vi "Charge_then_Discharge.vi"() -> ()   [LabVIEW 2020]
panel:
  out "PS error out":errorcluster
  out "PS Visa Out":refnum<visa-resource-name>
  in  "Discharge Current Cutoff":dbl
  in  "Discharge Current Setpoint (A)":dbl format="%#.6g"
  in  "Wait time":dbl
  in  "Batteryname":string
  in  "Charge Current Cutoff":dbl
  in  "Charge Current  Setpoint (A)":dbl format="%#.6g"
  in  "Battery Select":T1(ring)
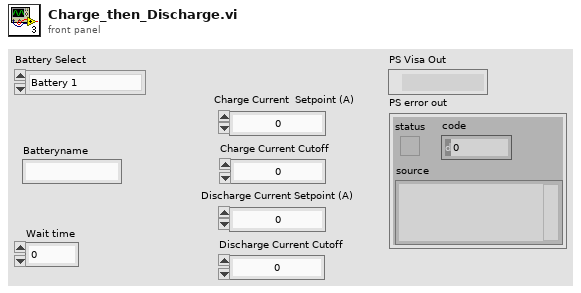
[diagram p1: front panel]
types:
  T1 = enum16{"Battery 1", "Battery 2", "Battery 3", "Battery 1&2", "Battery 1&3", "Battery 2&3", "Battery 1&2&3"}
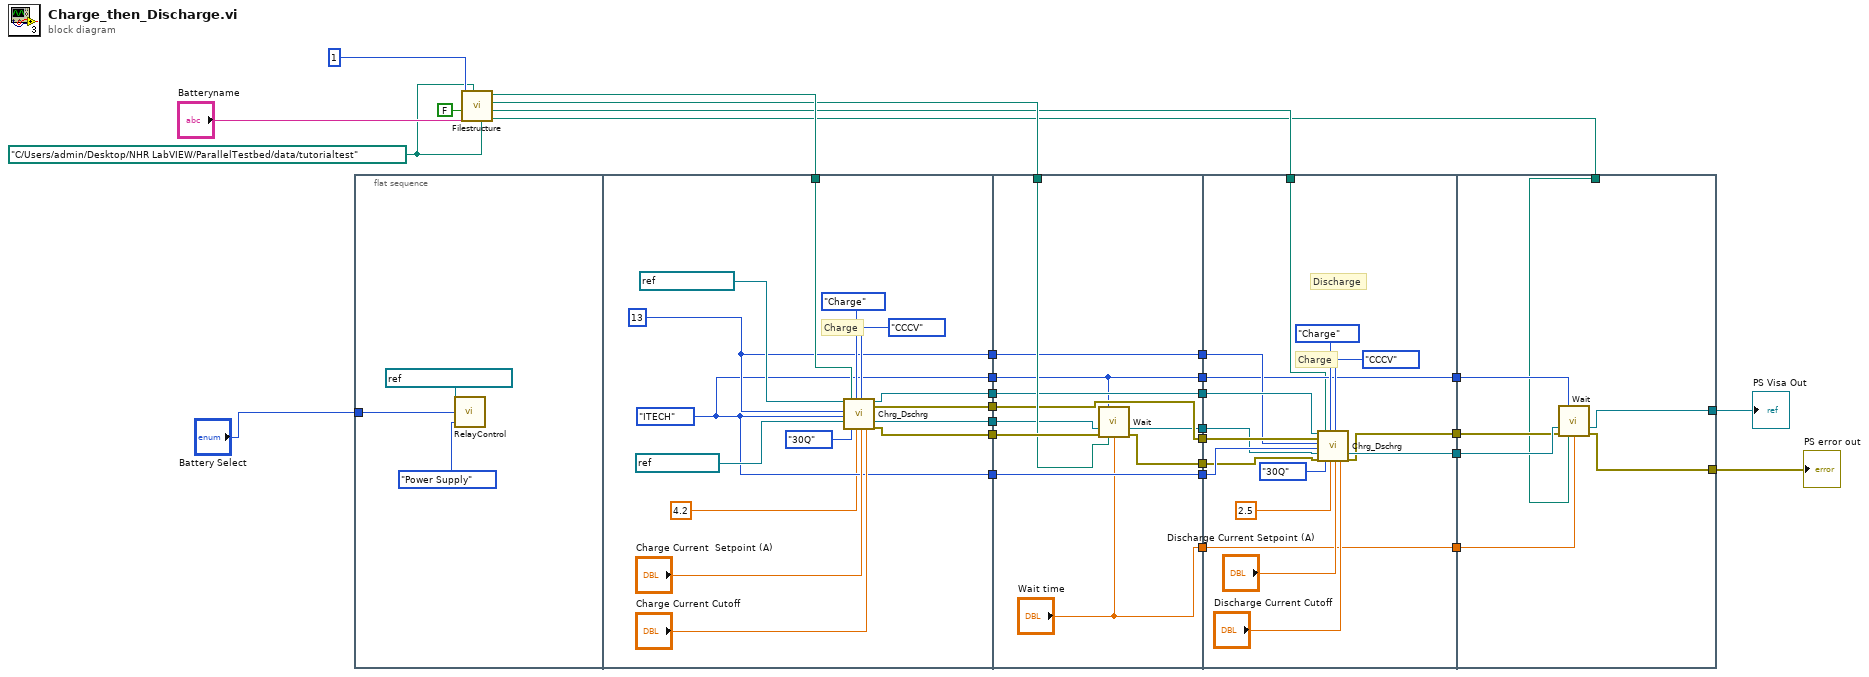
[diagram p0: block diagram]
diagram:
  w26 = path "C:/Users/admin/Desktop/NHR LabVIEW/ParallelTestbed/data/tutorialtest" ("Discharge filepath")
  n1 = flat-sequence {
    tunnel: "Battery Select" -> [w31]
    tunnel: w25 -> [w44]
    tunnel: [w41] -> w24
    tunnel: [w36] -> w23
    tunnel: [w38] -> w21
    tunnel: [w39] -> w19
    tunnel: [w37] -> w17
    tunnel: [w36] -> w15
    tunnel: [w35] -> w11
    tunnel: w24 -> [w59]
    tunnel: w23 -> [w50]
    tunnel: w22 -> [w58]
    tunnel: w21 -> [w57]
    tunnel: [w57] -> w20
    tunnel: w19 -> [w56]
    tunnel: [w56] -> w18
    tunnel: w17 -> [w55]
    tunnel: [w55] -> w16
    tunnel: w15 -> [w54]
    tunnel: [w54] -> w14
    tunnel: [w53] -> w13
    tunnel: [w52] -> w12
    tunnel: w11 -> [w51]
    tunnel: [w50] -> w8
    tunnel: ["Wait time"] -> w4
    tunnel: w20 -> [w73]
    tunnel: w18 -> [w72]
    tunnel: w16 -> [w71]
    tunnel: w14 -> [w70]
    tunnel: w13 -> [w69]
    tunnel: w12 -> [w68]
    tunnel: [w64] -> w10
    tunnel: [w63] -> w9
    tunnel: w8 -> [w62]
    tunnel: [w62] -> w7
    tunnel: w6 -> [w61]
    tunnel: w4 -> [w60]
    tunnel: [w60] -> w3
    tunnel: w10 -> [w83]
    tunnel: w9 -> [w82]
    tunnel: w7 -> [w81]
    tunnel: w5 -> [w80]
    tunnel: w3 -> [w79]
    tunnel: [w78] -> w2
    tunnel: [w77] -> w1
    frame #0 {
      n2 = call "RelayControl.vi"("NHR or Battery Analyzer"=enum16{"Battery Analyzer", "Power Supply"}."Power Supply", "Battery Select"=w31, "Relay Task"=refnum<k21> "PTestbedRelayTask") -> ()  [unwired: 2 in]
    }
    frame #1 {
      w36 = enum16{"NHR", "ITECH"}."ITECH" ("PS type")
      w37 = 13 ("#DAQ outputs (1-13)")
      # "Charge"
      n3 = call "Chrg_Dschrg.vi"("Data Task in"=refnum<k21> "PTesbedTask", "#DAQ outputs (1-13)"=w37, "PS type"=w36, "PS VISA in"=refnum<visa-resource-name> "ITECH-PS3", "CyclePath"=w44, "Battery Type"=enum16{"30Q", "40T"}."30Q", "Charge/discharge"=enum8{"Charge", "Discharge"}."Charge", "Charge/Discharge Voltage Setpoint"=4.2, "CC or CCCV"=enum16{"CC", "CCCV"}."CCCV", "Current Setpoint"="Charge Current  Setpoint (A)", "Current Cutoff"="Charge Current Cutoff") -> ("data task out"=w38:refnum<k21>, "data task error out"=w39:errorcluster, "VISA resource name out"=w35:refnum<visa-resource-name>, "NHR error out"=w41:errorcluster)  [unwired: 5 in]
    }
    frame #2 {
      n4 = call "Wait.vi"("PS type"=w50, "PS VISA in"=w51, "PS error in"=w59, "Wait Filepath"=w58, "Wait time"="Wait time") -> ("PS Visa Out"=w52:refnum<visa-resource-name>, "PS error out"=w53:errorcluster)  [unwired: 9 in]
    }
    frame #3 {
      # "Charge"
      # "Discharge"
      n5 = call "Chrg_Dschrg.vi"("Data Task in"=w73, "data task error in"=w72, "#DAQ outputs (1-13)"=w71, "PS type"=w70, "PS VISA in"=w68, "PS error in"=w69, "CyclePath"=w61, "Battery Type"=enum16{"30Q", "40T"}."30Q", "Charge/discharge"=enum8{"Charge", "Discharge"}."Charge", "Charge/Discharge Voltage Setpoint"=2.5, "CC or CCCV"=enum16{"CC", "CCCV"}."CCCV", "Current Setpoint"="Discharge Current Setpoint (A)", "Current Cutoff"="Discharge Current Cutoff") -> ("VISA resource name out"=w64:refnum<visa-resource-name>, "NHR error out"=w63:errorcluster)  [unwired: 3 in, 2 out]
    }
    frame #4 {
      n6 = call "Wait.vi"("PS type"=w81, "PS VISA in"=w83, "PS error in"=w82, "Wait Filepath"=w80, "Wait time"=w79) -> ("PS Visa Out"=w78:refnum<visa-resource-name>, "PS error out"=w77:errorcluster)  [unwired: 9 in]
    }
  }
  n7 = call "Filestructure.vi"("Discharge filepath"=w26, "Batteryname"="Batteryname", "Charge filepath"=w26, "In for loop"=FALSE, "Starting Cycle"=1) -> ("DischargeWaitPath"=w5:path, "DischargeCyclePath"=w6:path, "ChargeWaitPath"=w22:path, "ChargeCyclePath"=w25:path)  [unwired: 2 in, 1 out]
  "PS Visa Out" <- w2
  "PS error out" <- w1
